vi "RSZVB Set Slope.vi"(7 "Slope (0 dB/GHz)":dbl format="%^.3e", 8 "error in (no error)":errorcluster {"code" format="%.0x"}, 9 "Port (1)":i32=1, 10 "Channel (1)":i32=1, 11 "VISA session":refnum<visa-resource-name>) -> (0 "error out":errorcluster {"code" format="%.0x"}, 3 "dup VISA session":refnum<visa-resource-name>)   [LabVIEW 2011]
doc: "This VI defines a linear factor to modify the internal source power at port <Pt> as a VI of the stimulus frequency. \n\nNote(s):\n\n(1) The value can be set for frequency sweeps only.\n\nRemote-control command(s):\nSOURce<Ch>:POWer<Pt>[:LEVel][:IMMediate]:SLOPe <numeric_value>"
uses:
  _utility/RSZVB Global Data.vi
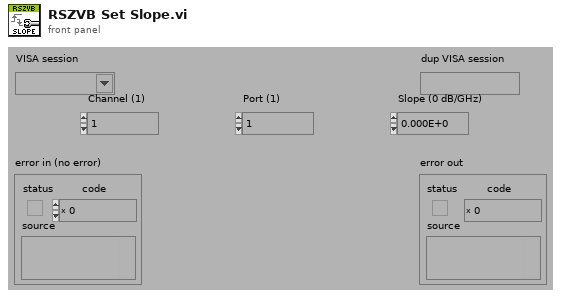
[diagram p1: front panel]
types:
  T1 = cluster{"Error Checking (T: On)":bool, "Installed Options":string[], "Data Valid?":bool, "Ports":i32, "Model":string[], "Option Checking (T: On)":bool}[]
  T2 = cluster{"Error Checking (T: On)":bool, "Installed Options":string[], "Data Valid?":bool, "Ports":i32, "Model":string[], "Option Checking (T: On)":bool}
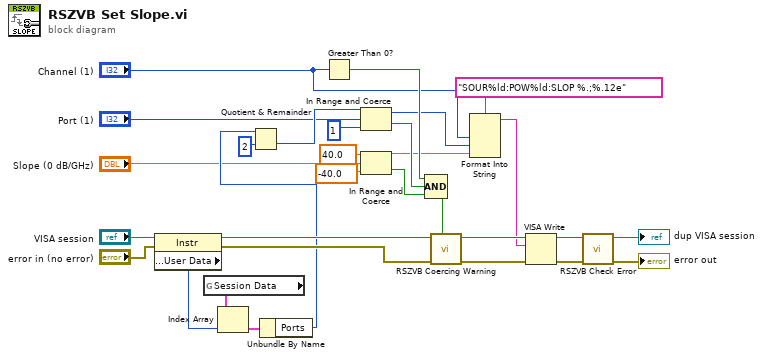
[diagram p0: block diagram]
diagram:
  n1 = property class="Instr"(reference="VISA session", error in="error in (no error)") -> (reference out=w18:refnum<visa-resource-name>, error out=w19:errorcluster, "General Settings:User Data"=w20:u32)
  n2 = global read "RSZVB Global Data.vi" "Session Data"() -> (w21:T1)
  n3 = Index Array(array=w21, index=w20) -> (element=w22:T2)
  n4 = Unbundle By Name(w22) -> ("Ports"=w11:i32)
  n5 = Quotient & Remainder(x=w11, y=2) -> (floor(x/y)=w13:i32)  [unwired: 1 out]
  n6 = Greater Than 0?(x="Channel (1)") -> (x > 0?=w23:bool)
  n7 = In Range and Coerce(upper limit=w13, x="Port (1)", lower limit=1) -> (coerced(x)=w12:i32, In Range?=w15:bool)
  n8 = In Range and Coerce(upper limit=40.0 ("lower limit"), x="Slope (0 dB/GHz)", lower limit=-40.0) -> (coerced(x)=w8:dbl, In Range?=w9:bool)
  n9 = Compound Arithmetic op=AND(w23, w15, w9) -> (w25:bool)
  n10 = call "RSZVB Coercing Warning.vi"("In Range?"=w25, "error in (no error)"=w19, "VISA session"=w18) -> ("error out"=w28:errorcluster, "dup VISA session"=w29:refnum<visa-resource-name>)  [unwired: 7 in]
  n11 = Format Into String(format string="SOUR%ld:POW%ld:SLOP %.;%.12e", "Channel (1)", w12, w8) -> (resulting string=w24:string)  [unwired: 2 in, 1 out]
  n12 = VISA Write(VISA resource name=w29, write buffer=w24, error in (no error)=w28) -> (VISA resource name out=w26:refnum<visa-resource-name>, error out=w27:errorcluster)  [unwired: 1 out]
  n13 = call "RSZVB Check Error.vi"("error in (no error)"=w27, "VISA session"=w26) -> ("error out"=→"error out":errorcluster, "dup VISA session"=→"dup VISA session":refnum<visa-resource-name>)  [unwired: 8 in]
